vi "OpenVLCPlayer.vi"(8 "error in":errorcluster, 9 "VLC executable path":path=path "C:/Program Files (x86)/VideoLAN/VLC/vlc.exe", 10 "VLC Port":u16=65123, 11 "VLC IP address":string="127.0.0.1") -> (0 "error out":errorcluster, 3 "Connection ID":refnum<k5>)   [LabVIEW 2015]
doc: "Open a VLC player instance with the RC (remote control) interface active. The other VLC VIs will be able to control the instance via a local TCP socket."
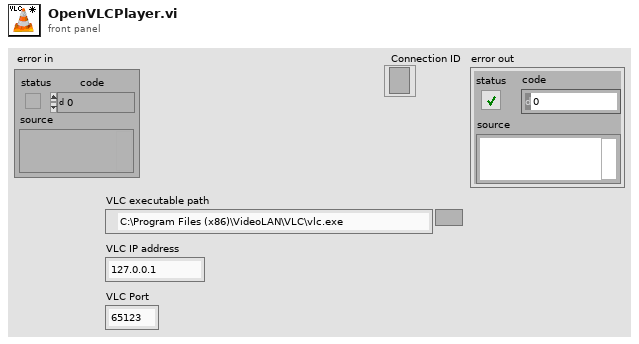
[diagram p1: front panel]
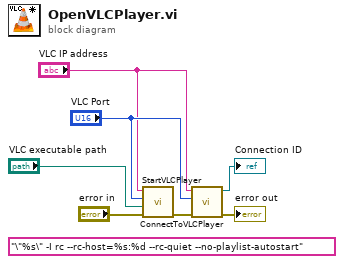
[diagram p0: block diagram]
diagram:
  (unwired) "\"%s\" -I rc --rc-host=%s:%d --rc-quiet --no-playlist-autostart" ("format string")
  n1 = call "StartVLCPlayer.vi"("error in"="error in", "VLC executable path"="VLC executable path", "VLC Port"="VLC Port", "VLC IP address"="VLC IP address") -> ("error out"=w7:errorcluster)  [unwired: 7 in]
  n2 = call "ConnectToVLCPlayer.vi"("error in"=w7, "VLC Port"="VLC Port", "VLC IP address"="VLC IP address") -> ("error out"=→"error out":errorcluster, "Connection ID"=→"Connection ID":refnum<k5>)  [unwired: 7 in]
